vi "uA_daq_Set_Opamp_Power_Supply_5.5VDC.vi"(8 "error in":errorcluster, 11 "USB DAQ":tag) -> (0 "error out":errorcluster)   [LabVIEW 2015]
uses:
  <vilib>/DAQmx/write.llb/DAQmx Write.vi
  <vilib>/DAQmx/write.llb/DAQmx Write (Analog DBL 1Chan 1Samp).vi
  <vilib>/DAQmx/create/channels.llb/DAQmx Create Channel (AO-Voltage-Basic).vi
  <vilib>/DAQmx/miscellaneous.llb/DAQmx Fill In Error Info.vi
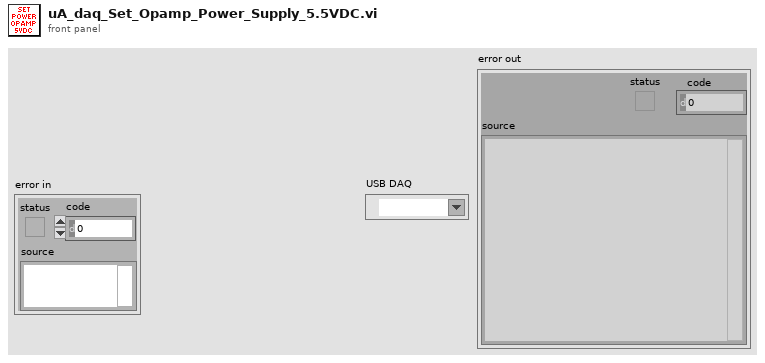
[diagram p1: front panel]
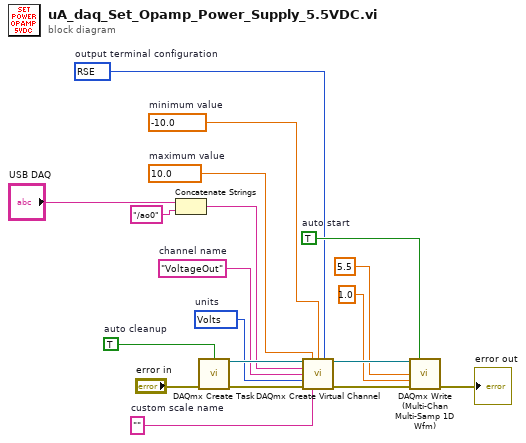
[diagram p0: block diagram]
diagram:
  w9 = 10083 items=["Default"=-1, "RSE"=10083, "Differential"=10106, "Pseudodifferential"=12529]  # output terminal configuration
  w10 = 10348 items=["Volts"=10348, "From Custom Scale"=10065]  # units
  w11 = "VoltageOut"  # channel name
  w12 = ""  # custom scale name
  w13 = -10.0  # minimum value
  w14 = 10.0  # maximum value
  w16 = TRUE  # auto cleanup
  w19 = TRUE  # auto start
  n1 = Concatenate Strings("USB DAQ", "/ao0" ("string")) -> (w2:string)
  n2 = call <vilib>:"DAQmx Create Task.vi"("auto cleanup"=w16, "error in"="error in") -> ("task out"=w15:refnum<k21>, "error out"=w17:errorcluster)  [unwired: 12 in]
  n3 = call-poly <vilib>:"DAQmx Create Virtual Channel.vi"("task in"=w15, "maximum value"=w14, "minimum value"=w13, "output terminal configuration"=w9, "physical channels"=w2, "name to assign"=w11, "units"=w10, "error in"=w17, "custom scale name"=w12) -> ("task out"=w8:refnum<k21>, "error out"=w5:errorcluster)  [unwired: 5 in]
  n4 = call-poly "DAQmx Write (Multi-Chan Multi-Samp 1D Wfm).vi"("task/channels in"=w8, "auto start"=w19, "data"=5.5, "timeout"=1.0, "error in"=w5) -> ("error out"=→"error out":errorcluster)  [unwired: 8 in, 2 out]
